vi "测试报告管理.vi"() -> ()   [LabVIEW 2010]
panel:
  out "查询语句":string
  in  "Row":dbl
  out "查询结果":string[][](table)
  in  "结束时间":timestamp
  in  "起始时间":timestamp
  in  "报告编号":string
  in  "btn_查询":bool
  in  "测试人员":string
  in  "测试地点":string
  in  "测试对象":string
  in  "单选_测试地点":bool
  in  "单选_测试人员":bool
  in  "单选_测试对象":bool
  in  "单选_测试报告编号":bool
  in  "单选_时间查询":bool
  in  "btn_返回":bool
  # "测试报告管理"
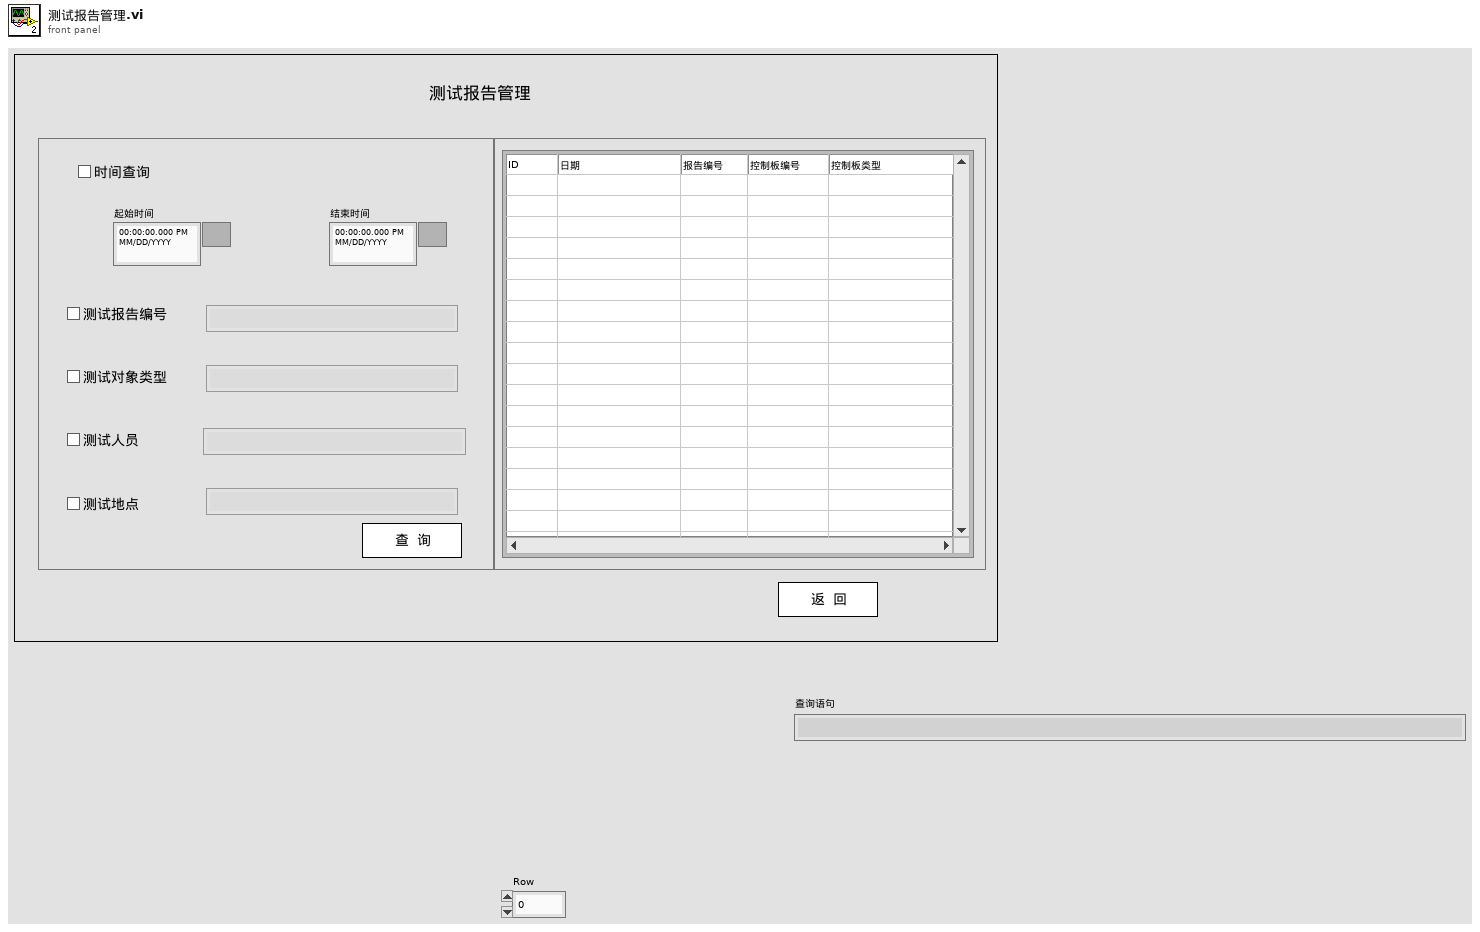
[diagram p1: front panel]
types:
  T1 = enum8{"Enabled", "Disabled", "Disabled and Grayed Out"}
  T2 = typedef "LVPoint32TypeDef.ctl" = cluster{"Horizontal":i32, "Vertical":i32}
  T3 = typedef "LVRowAndColumnTypeDef.ctl" = cluster{"Row":i32, "Column":i32}
  T4 = cluster{string, string, string, string, string, string, string, string, string, string, string}
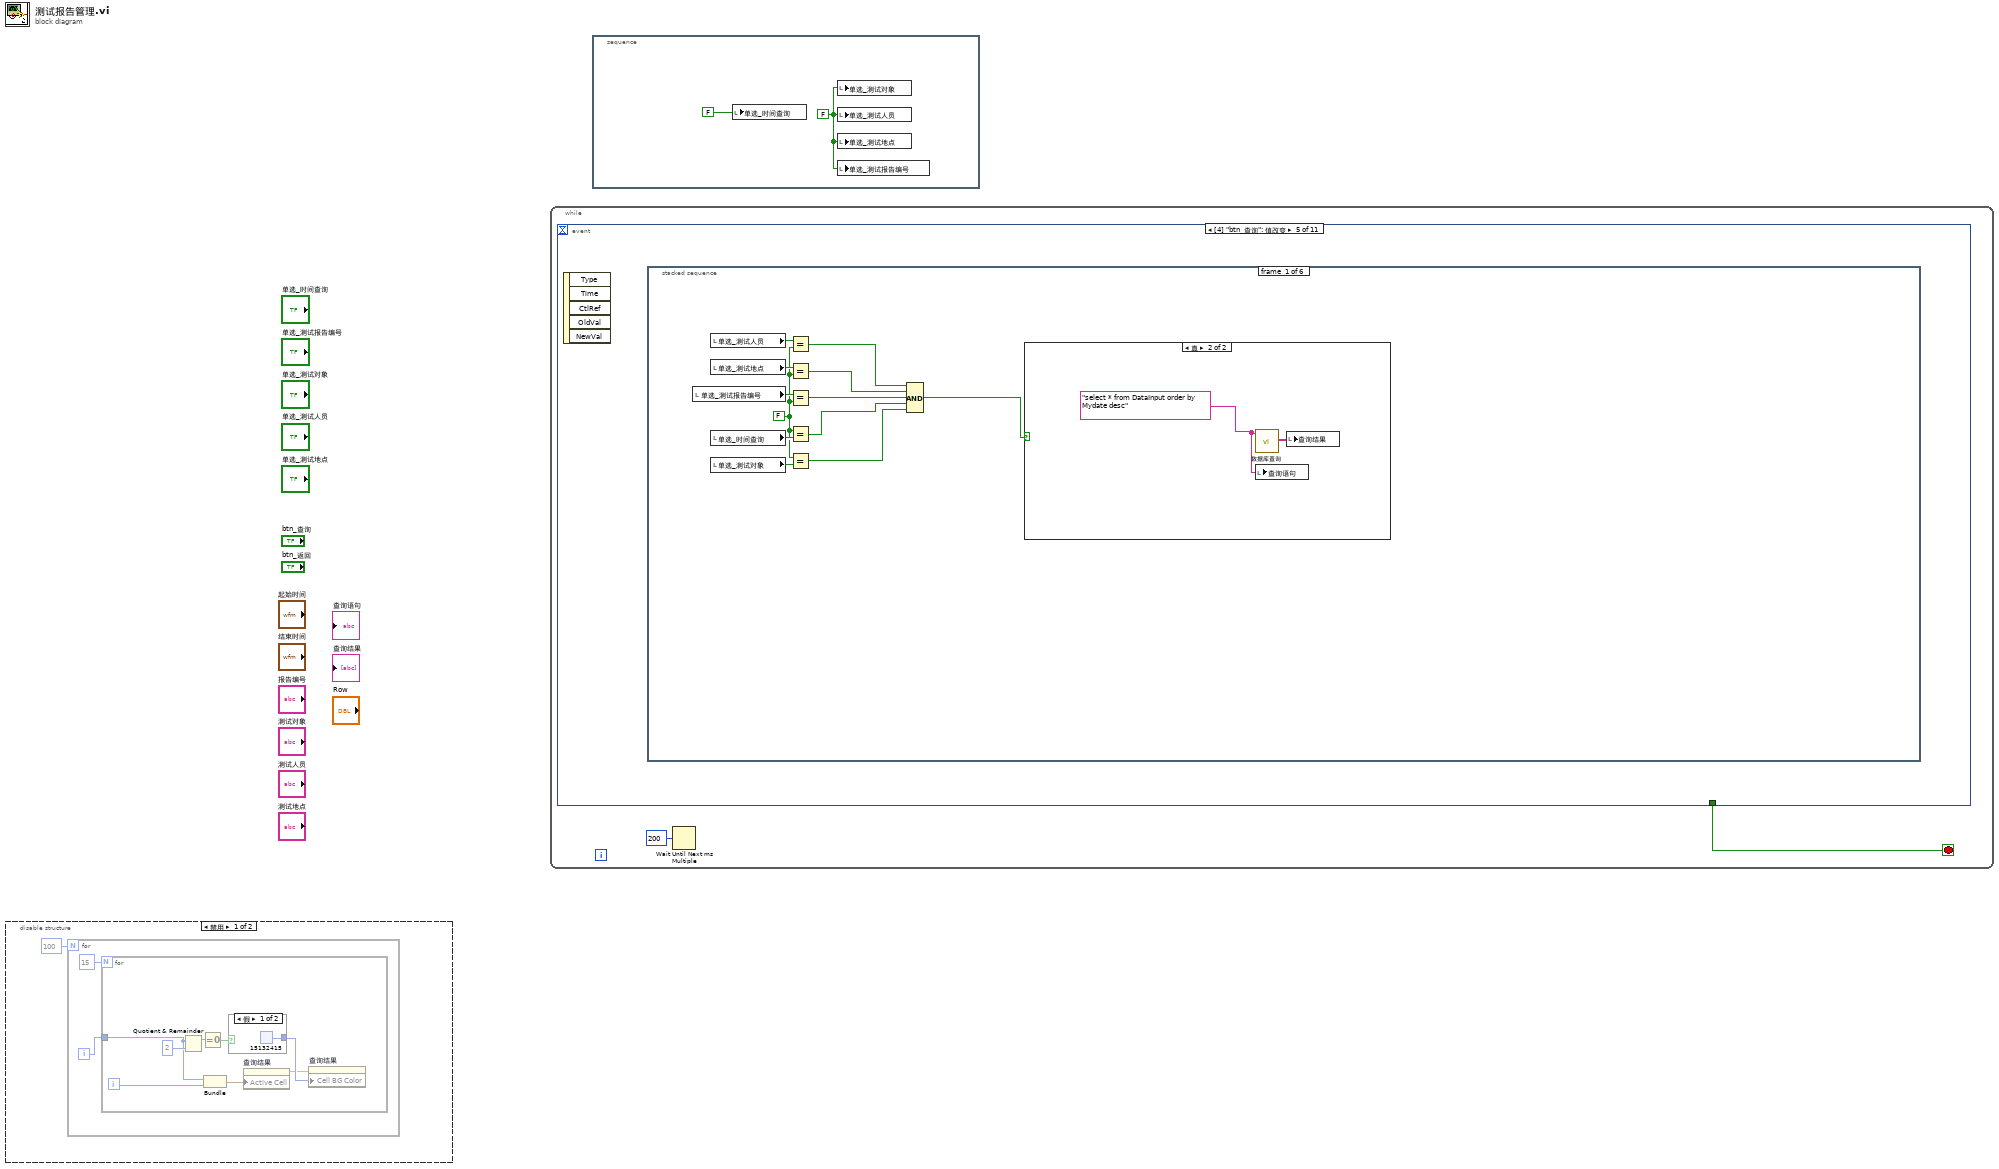
[diagram p0: block diagram]
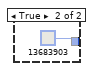
[diagram p2: hidden frame]
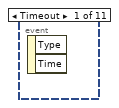
[diagram p4: hidden frame]
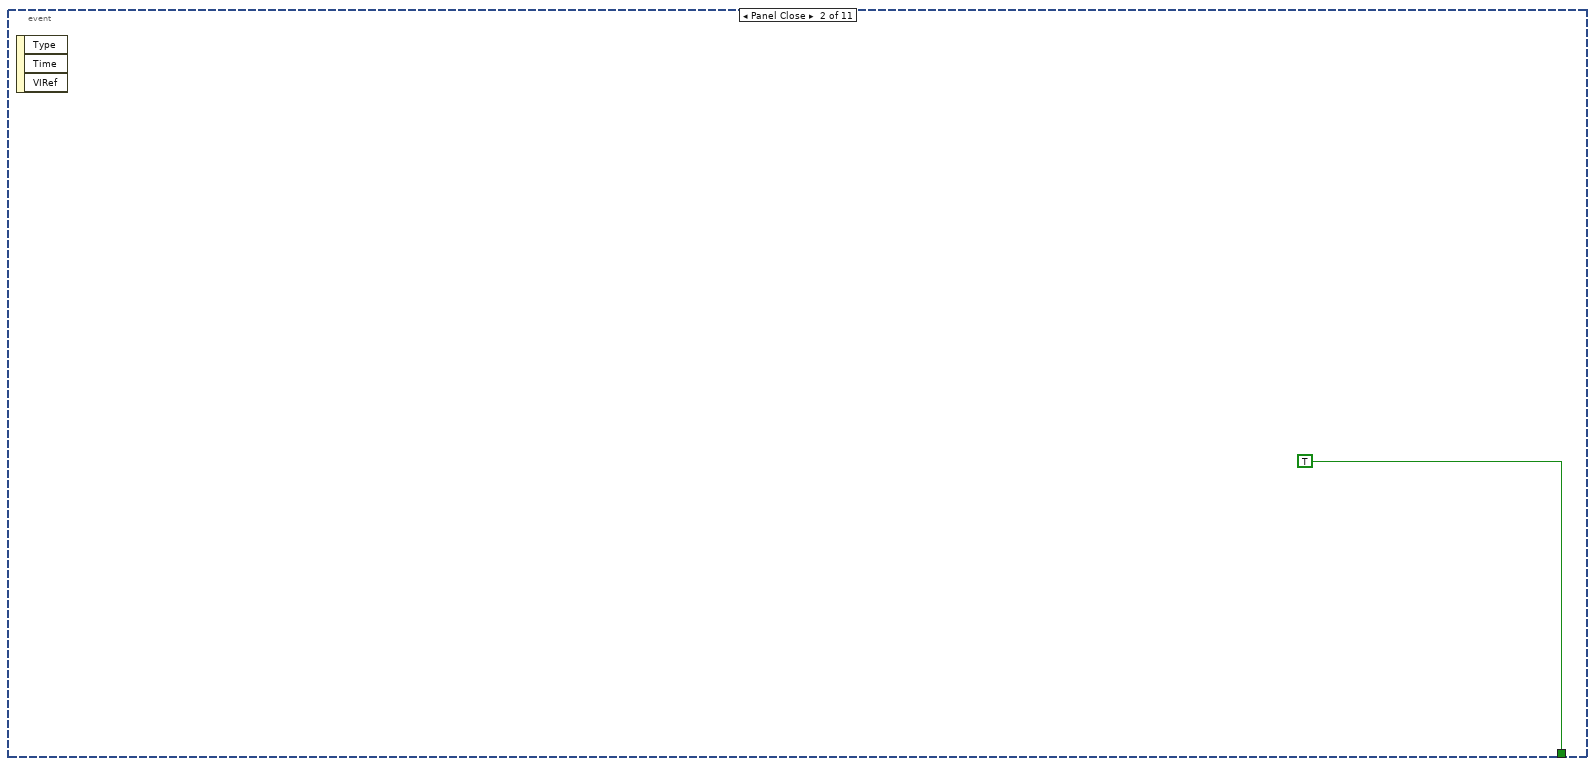
[diagram p5: hidden frame]
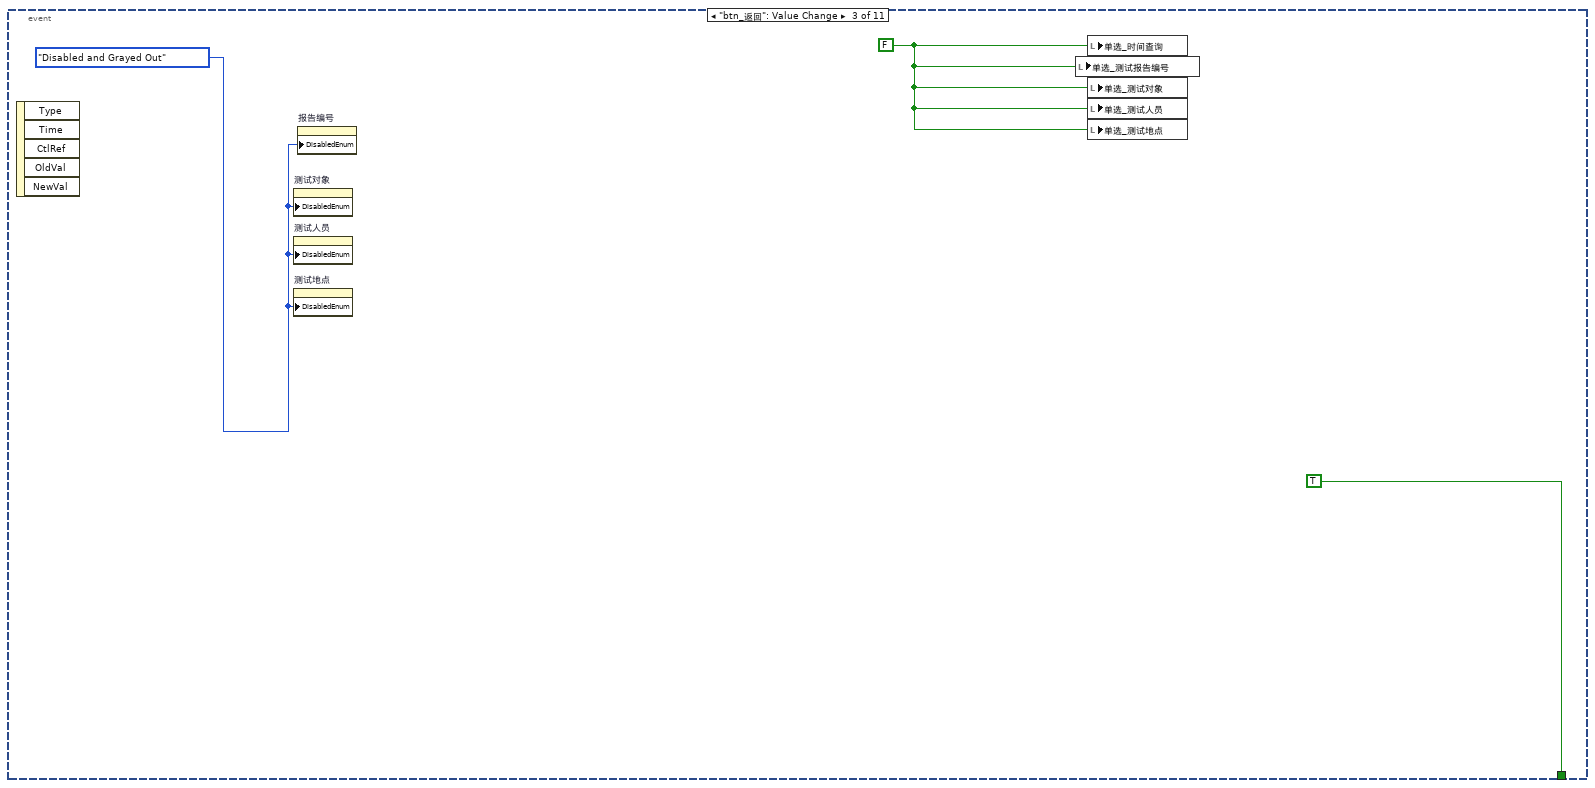
[diagram p6: hidden frame]
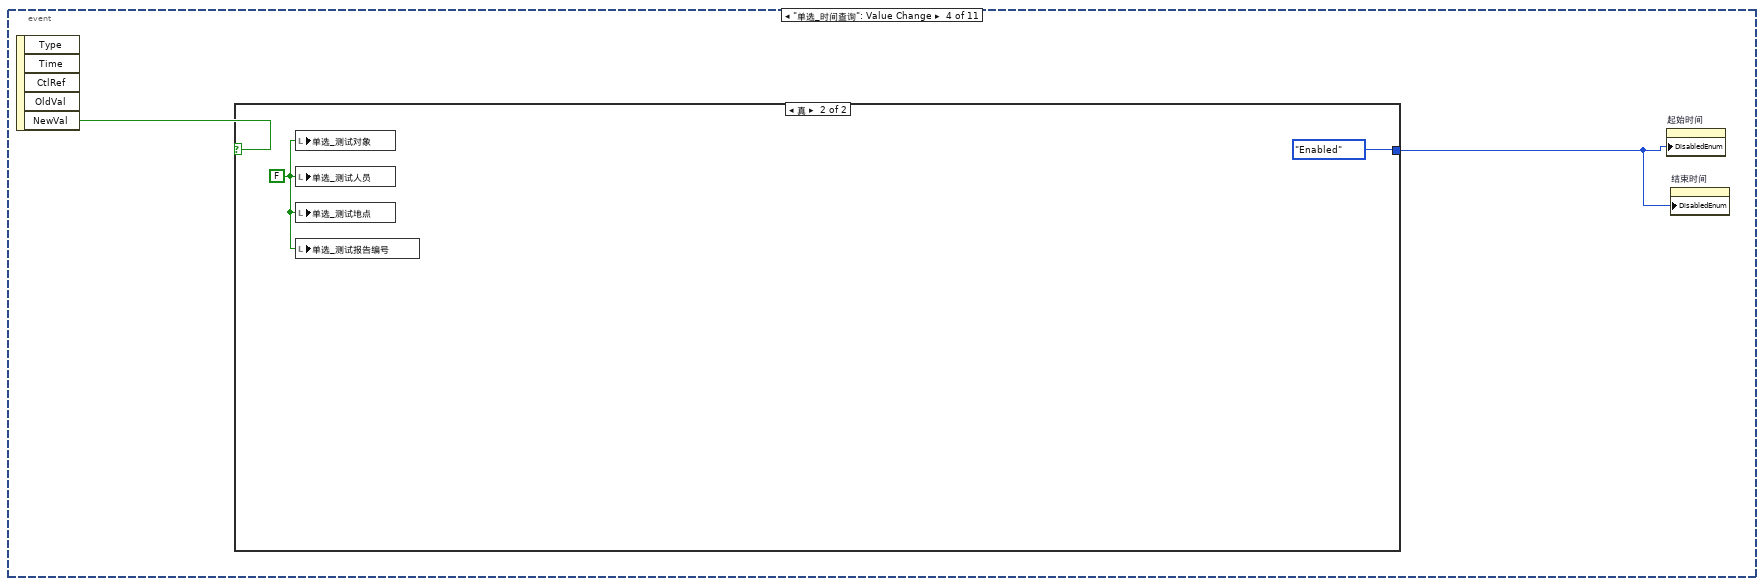
[diagram p7: hidden frame]
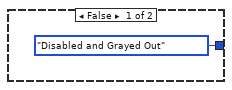
[diagram p8: hidden frame]
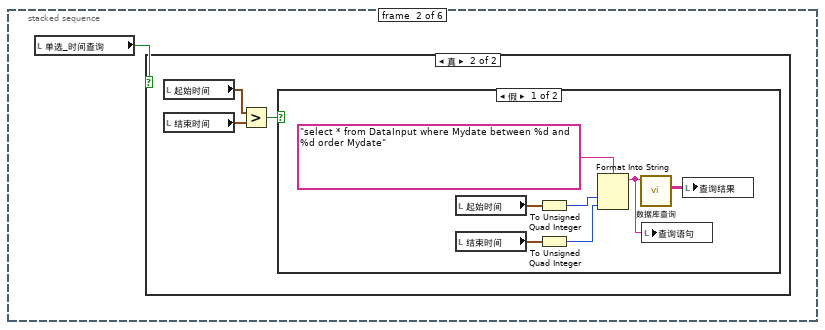
[diagram p10: hidden frame]
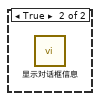
[diagram p12: hidden frame]
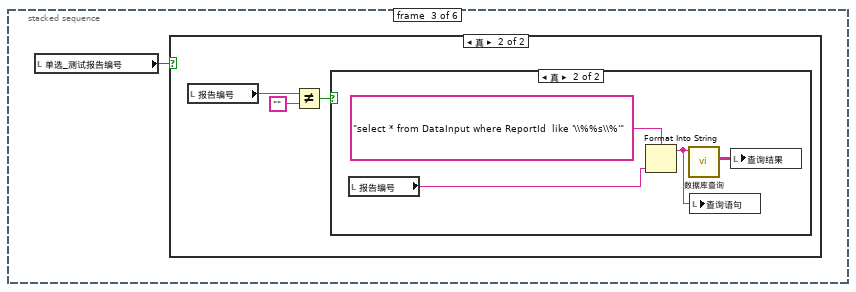
[diagram p13: hidden frame]
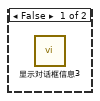
[diagram p15: hidden frame]
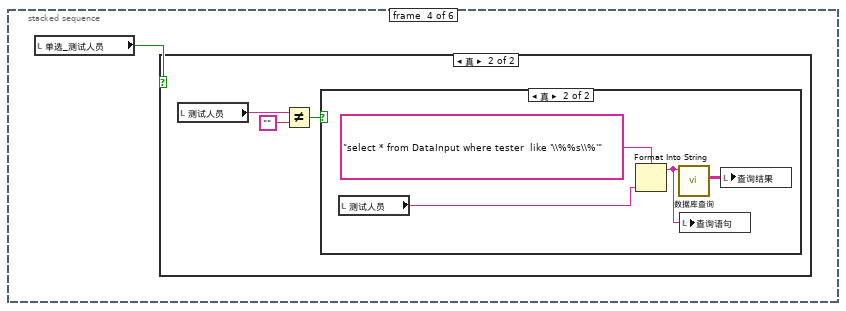
[diagram p16: hidden frame]
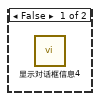
[diagram p18: hidden frame]
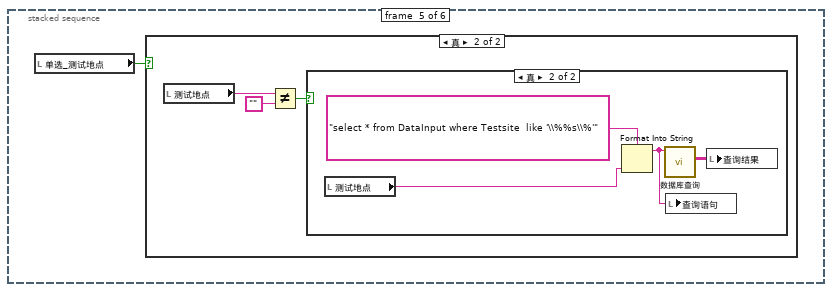
[diagram p19: hidden frame]
diagram:
  n1 = disable-structure shown="禁用" {
    frame Disabled {
      n2 = for {
        N: 100 -> [_]
        i -> [w2]
        n3 = for {
          N: 15 -> [_]
          tunnel: w2 -> [w4]
          i -> [w5]
          n4 = Quotient & Remainder(x=w4, y=2) -> (x-y*floor(x/y)=w7:i32)  [unwired: 1 out]
          n5 = Equal To 0?(x=w7) -> (x = 0?=w8:bool)
          n6 = Bundle(w4, w5) -> (w9:cluster{i32, i32})  [unwired: 1 in]
          n7 = case shown="假" w8 {
            tunnel: [u32 15132415 u32 13683903] -> w11
            frame False {
            }
            frame True {
            }
          }
          n8 = property on="查询结果" class="Tbl (严格)"("Active Cell"=w9) -> (error out=w6:errorcluster)  [unwired: 2 in, 1 out]
          n9 = property on="查询结果" class="Tbl (严格)"(error in=w6, "Cell BG Color"=w11) -> ()  [unwired: 1 in, 2 out]
        }
      }
    }
    frame Enabled {
    }
  }
  n10 = while {
    stop <- w15 stop-if-true
    n11 = event shown="[4] \"btn_查询\": 值改变" {
      selector: _ -> [_ _ _ _ _ _ _ _ _ _ _]
      dyn-events: _ -> [_ _ _ _ _ _ _ _ _ _ _]
      timeout: _ -> [_ _ _ _ _ _ _ _ _ _ _]
      tunnel: [_ TRUE TRUE _ _ _ _ _ _ _ _] -> w15
      event Timeout {
        n12 = event-data() -> ()  [unwired: 1 in, 2 out]
      }
      event Panel Close {
        n13 = event-data() -> ()  [unwired: 1 in, 3 out]
      }
      event "btn_返回": Value Change {
        w18 = FALSE ("单选_时间查询")
        w17 = T1."Disabled and Grayed Out" ("禁用")
        n14 = event-data() -> ()  [unwired: 1 in, 5 out]
        n15 = property on="测试对象" class="Str"("DisabledEnum"=w17) -> ()  [unwired: 2 in, 2 out]
        n16 = property on="测试人员" class="Str"("DisabledEnum"=w17) -> ()  [unwired: 2 in, 2 out]
        n17 = property on="测试地点" class="Str"("DisabledEnum"=w17) -> ()  [unwired: 2 in, 2 out]
        n18 = property on="报告编号" class="Str"("DisabledEnum"=w17) -> ()  [unwired: 2 in, 2 out]
        n19 = local write "单选_测试报告编号"(w18) -> ()
        n20 = local write "单选_时间查询"(w18) -> ()
        n21 = local write "单选_测试对象"(w18) -> ()
        n22 = local write "单选_测试人员"(w18) -> ()
        n23 = local write "单选_测试地点"(w18) -> ()
      }
      event "单选_时间查询": Value Change {
        n24 = event-data() -> ("NewVal"=w21:bool)  [unwired: 1 in, 4 out]
        n25 = case shown="真" w21 {
          tunnel: [T1."Disabled and Grayed Out" ("禁用") T1."Enabled" ("禁用")] -> w20
          frame False {
          }
          frame True {
            w23 = FALSE ("单选_测试报告编号")
            n26 = local write "单选_测试对象"(w23) -> ()
            n27 = local write "单选_测试人员"(w23) -> ()
            n28 = local write "单选_测试地点"(w23) -> ()
            n29 = local write "单选_测试报告编号"(w23) -> ()
          }
        }
        n30 = property on="起始时间" class="AbsTime (严格)"("DisabledEnum"=w20) -> ()  [unwired: 2 in, 2 out]
        n31 = property on="结束时间" class="AbsTime (严格)"("DisabledEnum"=w20) -> ()  [unwired: 2 in, 2 out]
      }
      event "btn_查询": Value Change {
        n32 = event-data() -> ()  [unwired: 1 in, 5 out]
        n33 = stacked-sequence {
          frame #0 {
            w31 = FALSE
            n34 = local read "单选_测试报告编号"() -> (w32:bool)
            n35 = local read "单选_测试人员"() -> (w34:bool)
            n36 = local read "单选_测试地点"() -> (w33:bool)
            n37 = local read "单选_时间查询"() -> (w35:bool)
            n38 = local read "单选_测试对象"() -> (w36:bool)
            n39 = Equal?(x=w34, y=w31) -> (x = y?=w30:bool)
            n40 = Equal?(x=w33, y=w31) -> (x = y?=w29:bool)
            n41 = Equal?(x=w32, y=w31) -> (x = y?=w28:bool)
            n42 = Equal?(x=w31, y=w35) -> (x = y?=w27:bool)
            n43 = Equal?(x=w31, y=w36) -> (x = y?=w26:bool)
            n44 = Compound Arithmetic op=AND(w30, w29, w28, w27, w26) -> (w25:bool)
            n45 = case shown="真" w25 {
              frame False {
              }
              frame True {
                w37 = "select * from DataInput order by Mydate desc" ("格式字符串")
                n46 = call "数据库查询.vi"("SQL语句"=w37) -> ("查询结果"=w38:string[][])  [unwired: 10 in]
                n47 = local write "查询语句"(w37) -> ()
                n48 = local write "查询结果"(w38) -> ()
              }
            }
          }
          frame #1 {
            n49 = local read "单选_时间查询"() -> (w39:bool)
            n50 = case shown="真" w39 {
              frame False {
              }
              frame True {
                n51 = local read "起始时间"() -> (w42:timestamp)
                n52 = local read "结束时间"() -> (w41:timestamp)
                n53 = Greater?(x=w42, y=w41) -> (0:w40:bool)
                n54 = case shown="假" w40 {
                  frame False {
                    n55 = local read "起始时间"() -> (w48:timestamp)
                    n56 = local read "结束时间"() -> (w49:timestamp)
                    n57 = To Unsigned Quad Integer(1:w48) -> (0:w47:u64)
                    n58 = To Unsigned Quad Integer(1:w49) -> (0:w46:u64)
                    n59 = Format Into String(format string="select * from DataInput where Mydate between %d and %d order Mydate" ("格式字符串"), w47, w46) -> (resulting string=w44:string)  [unwired: 2 in, 1 out]
                    n60 = call "数据库查询.vi"("SQL语句"=w44) -> ("查询结果"=w43:string[][])  [unwired: 10 in]
                    n61 = local write "查询语句"(w44) -> ()
                    n62 = local write "查询结果"(w43) -> ()
                  }
                  frame True {
                    n63 = call "显示对话框信息"() -> ()  [unwired: 10 in, 2 out]
                  }
                }
              }
            }
          }
          frame #2 {
            n64 = local read "单选_测试报告编号"() -> (w50:bool)
            n65 = case shown="真" w50 {
              frame False {
              }
              frame True {
                n66 = local read "报告编号"() -> (w53:string)
                n67 = Not Equal?(x=w53, y="") -> (x != y?=w51:bool)
                n68 = case shown="真" w51 {
                  frame False {
                    n69 = call "显示对话框信息3"() -> ()  [unwired: 10 in, 2 out]
                  }
                  frame True {
                    n70 = local read "报告编号"() -> (w54:string)
                    n71 = Format Into String(format string="select * from DataInput where ReportId  like '\\%%s\\%'" ("格式字符串"), w54) -> (resulting string=w56:string)  [unwired: 2 in, 1 out]
                    n72 = call "数据库查询.vi"("SQL语句"=w56) -> ("查询结果"=w55:string[][])  [unwired: 10 in]
                    n73 = local write "查询语句"(w56) -> ()
                    n74 = local write "查询结果"(w55) -> ()
                  }
                }
              }
            }
          }
          frame #3 {
            n75 = local read "单选_测试人员"() -> (w58:bool)
            n76 = case shown="真" w58 {
              frame False {
              }
              frame True {
                n77 = local read "测试人员"() -> (w60:string)
                n78 = Not Equal?(x=w60, y="") -> (x != y?=w59:bool)
                n79 = case shown="真" w59 {
                  frame False {
                    n80 = call "显示对话框信息4"() -> ()  [unwired: 10 in, 2 out]
                  }
                  frame True {
                    n81 = local read "测试人员"() -> (w62:string)
                    n82 = Format Into String(format string="select * from DataInput where tester  like '\\%%s\\%'" ("格式字符串"), w62) -> (resulting string=w64:string)  [unwired: 2 in, 1 out]
                    n83 = call "数据库查询.vi"("SQL语句"=w64) -> ("查询结果"=w63:string[][])  [unwired: 10 in]
                    n84 = local write "查询语句"(w64) -> ()
                    n85 = local write "查询结果"(w63) -> ()
                  }
                }
              }
            }
          }
          frame #4 {
            n86 = local read "单选_测试地点"() -> (w66:bool)
            n87 = case shown="真" w66 {
              frame False {
              }
              frame True {
                n88 = local read "测试地点"() -> (w68:string)
                n89 = Not Equal?(x=w68, y="") -> (x != y?=w67:bool)
                n90 = case shown="真" w67 {
                  frame False {
                    n91 = call "显示对话框信息5"() -> ()  [unwired: 10 in, 2 out]
                  }
                  frame True {
                    n92 = local read "测试地点"() -> (w70:string)
                    n93 = Format Into String(format string="select * from DataInput where Testsite  like '\\%%s\\%'" ("格式字符串"), w70) -> (resulting string=w72:string)  [unwired: 2 in, 1 out]
                    n94 = call "数据库查询.vi"("SQL语句"=w72) -> ("查询结果"=w71:string[][])  [unwired: 10 in]
                    n95 = local write "查询语句"(w72) -> ()
                    n96 = local write "查询结果"(w71) -> ()
                  }
                }
              }
            }
          }
          frame #5 {
            n97 = local read "单选_测试对象"() -> (w74:bool)
            n98 = case shown="真" w74 {
              frame False {
              }
              frame True {
                n99 = local read "测试对象"() -> (w76:string)
                n100 = Not Equal?(x=w76, y="") -> (x != y?=w75:bool)
                n101 = case shown="真" w75 {
                  frame False {
                    n102 = call "显示对话框信息6"() -> ()  [unwired: 10 in, 2 out]
                  }
                  frame True {
                    n103 = local read "测试对象"() -> (w78:string)
                    n104 = Format Into String(format string="select * from DataInput where ControlboardType  like '\\%%s\\%'" ("格式字符串"), w78) -> (resulting string=w80:string)  [unwired: 2 in, 1 out]
                    n105 = local write "查询语句"(w80) -> ()
                    n106 = call "数据库查询.vi"("SQL语句"=w80) -> ("查询结果"=w79:string[][])  [unwired: 10 in]
                    n107 = local write "查询结果"(w79) -> ()
                  }
                }
              }
            }
          }
        }
      }
      event "查询结果": Shortcut Menu Activation? {
        n108 = event-data() -> ("Coords"=w83:T2)  [unwired: 1 in, 5 out]
        n109 = invoke on="查询结果" class="Tbl (严格)" method="Point To Row Column"("Point"=w83) -> ("CellPosition"=w86:T3)  [unwired: 5 in, 5 out]
        n110 = Unbundle(w86) -> ("Row"=w82:i32)  [unwired: 1 out]
        n111 = Equal?(x=w82, y=-1) -> (x = y?=w84:bool)
        n112 = local write "Row"(w82) -> ()
        n113 = event-data("Discard?"=w84) -> ()  [unwired: 1 in, 1 out]
      }
      event "查询结果": Shortcut Menu Selection (User) {
        n114 = event-data() -> ("ItemTag"=w87:string)  [unwired: 1 in, 6 out]
        n115 = case shown="\"生成报告\", 默认" w87 {
          frame "生成报告", Default {
            n116 = local read "查询结果"() -> (w114:string[][])
            n117 = local read "Row"() -> (w113:dbl)
            n118 = Index Array(array=w114, index (row)=w113) -> (element=w112:string[])  [unwired: 1 in]
            n119 = Index Array(array=w112, index #1=1, index #2=2, index #3=3, index #4=4, index #5=5, index #6=6, index #7=7, index #8=8, index #9=9, index #10=10, index #11=11) -> (element #1=w111:string, element #2=w110:string, element #3=w109:string, element #4=w108:string, element #5=w107:string, element #6=w106:string, element #7=w105:string, element #8=w104:string, element #9=w92:string, element #10=w91:string, element #11=w90:string)
            n120 = Bundle(w111, w110, w109, w108, w107, w106, w105, w104, w92, w91, w90) -> (w89:T4)  [unwired: 1 in]
            n121 = call "生成报告.vi"("打印?"=FALSE, "输出簇"=w89) -> ()  [unwired: 9 in]
          }
          frame "打印" {
            n122 = local read "查询结果"() -> (w141:string[][])
            n123 = local read "Row"() -> (w140:dbl)
            n124 = Index Array(array=w141, index (row)=w140) -> (element=w139:string[])  [unwired: 1 in]
            n125 = Index Array(array=w139, index #1=1, index #2=2, index #3=3, index #4=4, index #5=5, index #6=6, index #7=7, index #8=8, index #9=9, index #10=10, index #11=11) -> (element #1=w138:string, element #2=w137:string, element #3=w136:string, element #4=w135:string, element #5=w134:string, element #6=w133:string, element #7=w132:string, element #8=w131:string, element #9=w119:string, element #10=w118:string, element #11=w117:string)
            n126 = Bundle(w138, w137, w136, w135, w134, w133, w132, w131, w119, w118, w117) -> (w116:T4)  [unwired: 1 in]
            n127 = call "报告打印.vi"("输出簇"=w116, "打印?"=TRUE) -> ()  [unwired: 10 in]
          }
          frame "删除" {
            n128 = local read "查询结果"() -> (w143:string[][])
            n129 = local read "Row"() -> (w144:dbl)
            n130 = Index Array(array=w143, index (row)=w144, index (col)=0 ("禁用的索引 (列)")) -> (element=w146:string)
            n131 = Decimal String To Number(string=w146) -> (number=w142:i32)  [unwired: 2 in, 1 out]
            n132 = Format Into String(format string="确认要删除本条记录么？\n报告ID：%d" ("消息"), w142) -> (resulting string=w148:string)  [unwired: 2 in, 1 out]
            n133 = Two Button Dialog(message=w148) -> (T button?=w147:bool)  [unwired: 2 in]
            n134 = case shown="真" w147 {
              tunnel: w142 -> [_ w150]
              frame False {
              }
              frame True {
                n135 = stacked-sequence {
                  tunnel: w150 -> [w151 _ _]
                  frame #0 {
                    n136 = call "删除一条记录.vi"("ID"=w151) -> ()  [unwired: 11 in]
                  }
                  frame #1 {
                    n137 = Wait (ms)(milliseconds to wait=u32 1000 ("等待时间（毫秒）")) -> ()  [unwired: 1 out]
                  }
                  frame #2 {
                    n138 = local read "查询语句"() -> (w153:string)
                    n139 = call "数据库查询.vi"("SQL语句"=w153) -> ("查询结果"=w154:string[][])  [unwired: 10 in]
                    n140 = local write "查询结果"(w154) -> ()
                  }
                }
              }
            }
          }
        }
      }
      event "单选_测试报告编号": Value Change {
        n141 = event-data() -> ("NewVal"=w156:bool)  [unwired: 1 in, 4 out]
        n142 = case shown="真" w156 {
          tunnel: [T1."Disabled and Grayed Out" ("禁用") T1."Enabled" ("禁用")] -> w155
          frame False {
          }
          frame True {
            w158 = FALSE ("单选_测试报告编号")
            n143 = local write "单选_测试对象"(w158) -> ()
            n144 = local write "单选_测试人员"(w158) -> ()
            n145 = local write "单选_测试地点"(w158) -> ()
            n146 = local write "单选_时间查询"(w158) -> ()
          }
        }
        n147 = property on="报告编号" class="Str"("DisabledEnum"=w155) -> ()  [unwired: 2 in, 2 out]
      }
      event "单选_测试对象": Value Change {
        n148 = event-data() -> ("NewVal"=w161:bool)  [unwired: 1 in, 4 out]
        n149 = case shown="真" w161 {
          tunnel: [T1."Disabled and Grayed Out" ("禁用") T1."Enabled" ("禁用")] -> w160
          frame False {
          }
          frame True {
            w163 = FALSE ("单选_测试报告编号")
            n150 = local write "单选_时间查询"(w163) -> ()
            n151 = local write "单选_测试人员"(w163) -> ()
            n152 = local write "单选_测试地点"(w163) -> ()
            n153 = local write "单选_测试报告编号"(w163) -> ()
          }
        }
        n154 = property on="测试对象" class="Str"("DisabledEnum"=w160) -> ()  [unwired: 2 in, 2 out]
      }
      event "单选_测试人员": Value Change {
        n155 = event-data() -> ("NewVal"=w166:bool)  [unwired: 1 in, 4 out]
        n156 = case shown="真" w166 {
          tunnel: [T1."Disabled and Grayed Out" ("禁用") T1."Enabled" ("禁用")] -> w165
          frame False {
          }
          frame True {
            w168 = FALSE ("单选_测试报告编号")
            n157 = local write "单选_测试对象"(w168) -> ()
            n158 = local write "单选_时间查询"(w168) -> ()
            n159 = local write "单选_测试地点"(w168) -> ()
            n160 = local write "单选_测试报告编号"(w168) -> ()
          }
        }
        n161 = property on="测试人员" class="Str"("DisabledEnum"=w165) -> ()  [unwired: 2 in, 2 out]
      }
      event "单选_测试地点": Value Change {
        n162 = event-data() -> ("NewVal"=w171:bool)  [unwired: 1 in, 4 out]
        n163 = case shown="真" w171 {
          tunnel: [T1."Disabled and Grayed Out" ("禁用") T1."Enabled" ("禁用")] -> w170
          frame False {
          }
          frame True {
            w173 = FALSE ("单选_测试报告编号")
            n164 = local write "单选_测试对象"(w173) -> ()
            n165 = local write "单选_测试人员"(w173) -> ()
            n166 = local write "单选_时间查询"(w173) -> ()
            n167 = local write "单选_测试报告编号"(w173) -> ()
          }
        }
        n168 = property on="测试地点" class="Str"("DisabledEnum"=w170) -> ()  [unwired: 2 in, 2 out]
      }
    }
    n169 = Wait Until Next ms Multiple(millisecond multiple=u32 200 ("毫秒倍数")) -> ()  [unwired: 1 out]
  }
  n170 = stacked-sequence {
    frame #0 {
      w175 = FALSE ("单选_测试报告编号")
      n171 = local write "单选_时间查询"(FALSE ("单选_时间查询")) -> ()
      n172 = local write "单选_测试对象"(w175) -> ()
      n173 = local write "单选_测试人员"(w175) -> ()
      n174 = local write "单选_测试地点"(w175) -> ()
      n175 = local write "单选_测试报告编号"(w175) -> ()
    }
  }
